vi "CONTROL POR VOZ_COVID_19.vi"() -> ()   [LabVIEW 2019]
panel:
  out "Boolean 3":bool
  out "Boolean 2":bool
  out "Boolean":bool
  in  "Phrases":i32(listbox)
  out "Score":dbl
  in  "Exit":bool
  out "Command":string
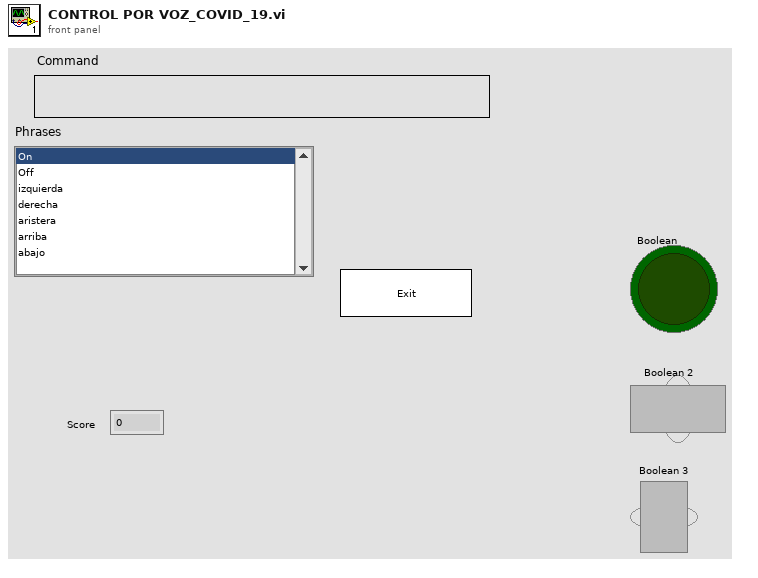
[diagram p1: front panel]
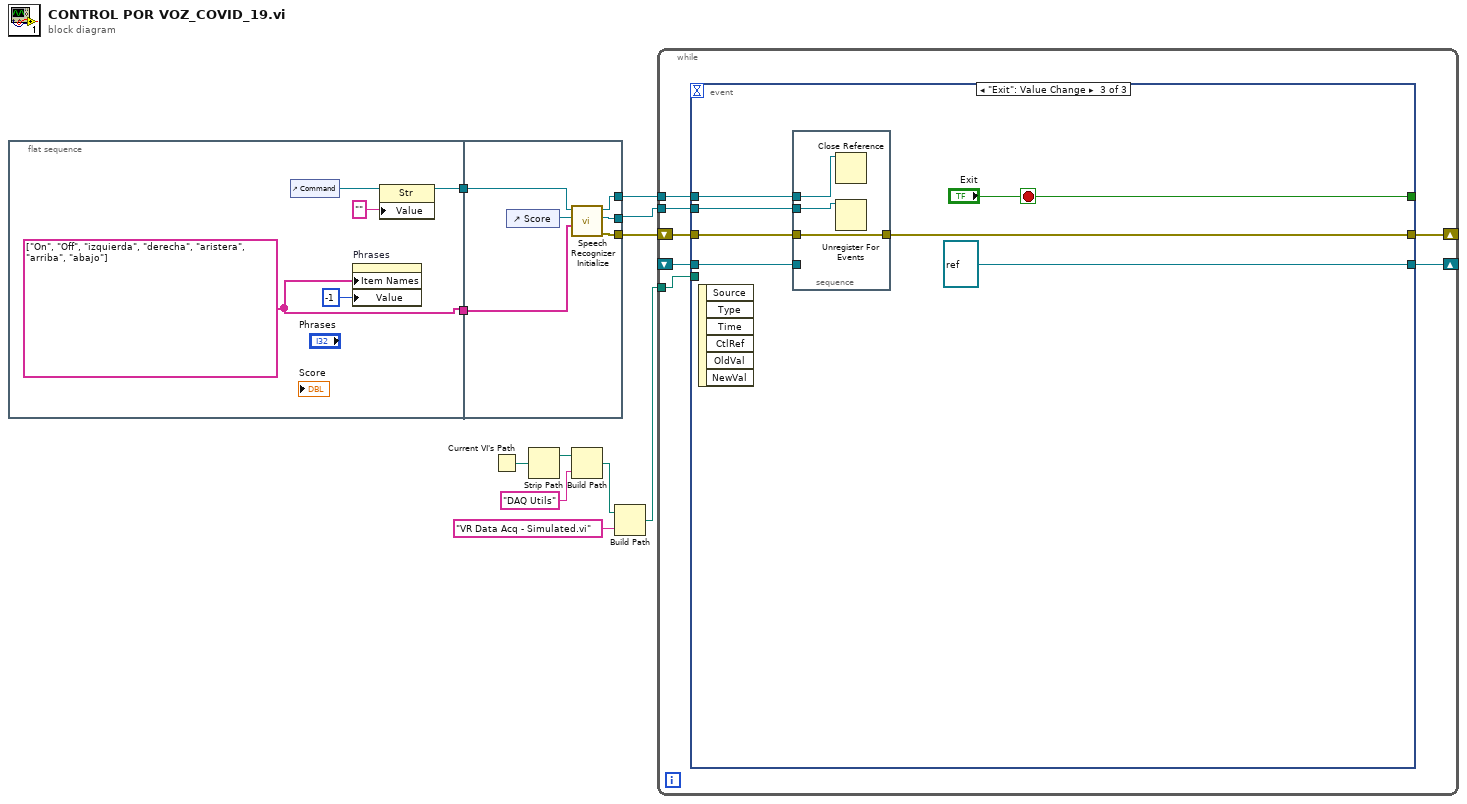
[diagram p0: block diagram]
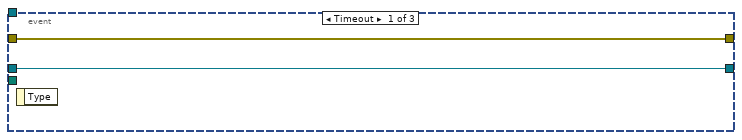
[diagram p2: hidden frame]
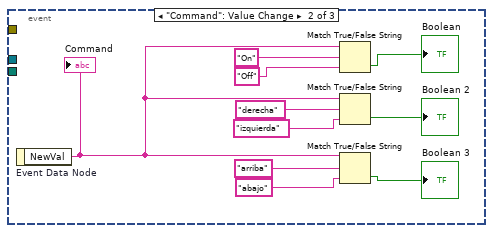
[diagram p3: hidden frame]
diagram:
  n1 = flat-sequence {
    tunnel: [w12] -> w11
    tunnel: [w14] -> w10
    tunnel: [w22] -> w9
    tunnel: [w21] -> w8
    tunnel: [w20] -> w7
    tunnel: w11 -> [w19]
    tunnel: w10 -> [w17]
    frame #0 {
      w12 = string[] ["On", "Off", "izquierda", "derecha", "aristera", "arriba", "abajo"] ("Item Names")
      n2 = control-ref of="Command"() -> (w16:refnum<vi>)
      n3 = property on="Phrases" class="LstBox (strict)"("Item Names"=w12, "Value"=-1) -> ()  [unwired: 2 in, 2 out]
      n4 = property class="Str"(reference=w16, "Value"="") -> (reference out=w14:refnum<vi>)  [unwired: 1 in, 1 out]
    }
    frame #1 {
      n5 = control-ref of="Score"() -> (w18:refnum<vi>)
      n6 = call "Speech Recognizer Initialize.vi"("String[] phrases"=w19, "Score"=w18, "Text"=w17) -> ("error out"=w22:errorcluster, "Event Callback"=w21:refnum<k27>, "reference"=w20:refnum<k24>)  [unwired: 6 out]
    }
  }
  n7 = Current VI's Path() -> (path=w2:path)
  n8 = Strip Path(path=w2) -> (stripped path=w1:path)  [unwired: 1 out]
  n9 = Build Path(base path=w1, name or relative path="DAQ Utils") -> (appended path=w5:path)
  n10 = Build Path(base path=w5, name or relative path="VR Data Acq - Simulated.vi") -> (appended path=w3:path)
  n11 = while {
    shift-right: [w28] -> _
    shift-left: w9 -> [w30]
    tunnel: w8 -> [w27]
    tunnel: w7 -> [w26]
    tunnel: w3 -> [w25]
    shift-right: [w24] -> _
    shift-left: _ -> [w23]
    stop <- w29 stop-if-true
    n12 = event shown="[2] \"Exit\": Value Change" {
      selector: _ -> [_ _ _]
      dyn-events: _ -> [_ _ _]
      timeout: _ -> [_ _ _]
      tunnel: w30 -> [w32 _ w48]
      tunnel: [_ _ "Exit"] -> w29
      tunnel: [w32 _ w43] -> w28
      tunnel: w27 -> [_ _ w47]
      tunnel: w26 -> [_ _ w46]
      tunnel: w25 -> [_ _ _]
      tunnel: [w31 _ refnum<vi> refnum ("vi reference")] -> w24
      tunnel: w23 -> [w31 _ w45]
      event Timeout {
        n13 = event-data() -> ()  [unwired: 2 out]
      }
      event "Command": Value Change {
        n14 = event-data "Event Data Node"() -> ("NewVal"=w42:string)  [unwired: 1 out]
        "Command" <- w42
        n15 = Match True/False String(2:"Off", 3:"On", 4:w42) -> (0:→"Boolean":bool)  [unwired: 1 out]
        n16 = Match True/False String(2:"izquierda", 3:"derecha", 4:w42) -> (0:→"Boolean 2":bool)  [unwired: 1 out]
        n17 = Match True/False String(2:"abajo", 3:"arriba", 4:w42) -> (0:→"Boolean 3":bool)  [unwired: 1 out]
      }
      event "Exit": Value Change {
        n18 = event-data() -> ()  [unwired: 7 out]
        n19 = stacked-sequence {
          tunnel: w48 -> [w50]
          tunnel: w47 -> [w52]
          tunnel: w46 -> [w51]
          tunnel: w45 -> [_]
          tunnel: [w50] -> w43
          frame #0 {
            n20 = Close Reference(reference=w51) -> ()  [unwired: 1 in, 1 out]
            n21 = Unregister For Events(event registration refnum=w52) -> ()  [unwired: 1 in, 1 out]
          }
        }
      }
    }
  }
